vi "niRFUtil FWK Get Driver Version.vi"(8 "error in (no error)":errorcluster, 11 "Registry Key":string[](array[string])=["SOFTWARE\\National Instruments\\NI-RFSA\\Run-Time", "SOFTWARE\\National Instruments\\VST\\NI-RFSA Support\\Current Version", "SOFTWARE\\National Instruments\\VST20\\NI-RFSA Support\\Current Version"]) -> (0 "error out":errorcluster, 1 "Major Version":i32, 2 "VersionString":string, 3 "Version":string, 4 "Minor Version":i32)   [LabVIEW 2015, in "niRFUtil.lvlib"]
uses:
  niRFUtil.lvlib
  <vilib>/registry/registry.llb/Registry RtKey.ctl
  <vilib>/registry/registry.llb/Registry SAM.ctl
  <vilib>/registry/registry.llb/Read Registry Value Simple STR.vi
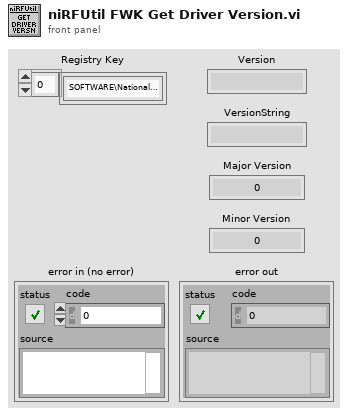
[diagram p1: front panel]
types:
  T1 = typedef "Registry SAM.ctl" = enum32{"KEY_QUERY_VALUE", "KEY_SET_VALUE", "KEY_CREATE_SUB_KEY", "KEY_ENUMERATE_SUB_KEYS", "KEY_NOTIFY", "KEY_CREATE_LINK", "KEY_READ", "KEY_WRITE", "KEY_ALL_ACCESS", "KEY_READ | KEY_WRITE"}
  T2 = typedef "Registry RtKey.ctl" = enum32{"HKEY_CLASSES_ROOT", "HKEY_CURRENT_USER", "HKEY_LOCAL_MACHINE", "HKEY_USERS", "HKEY_PERFORMANCE_DATA", "HKEY_CURRENT_CONFIG", "HKEY_DYN_DATA"}
  T3 = typedef "Registry refnum.ctl" = refnum<k1>
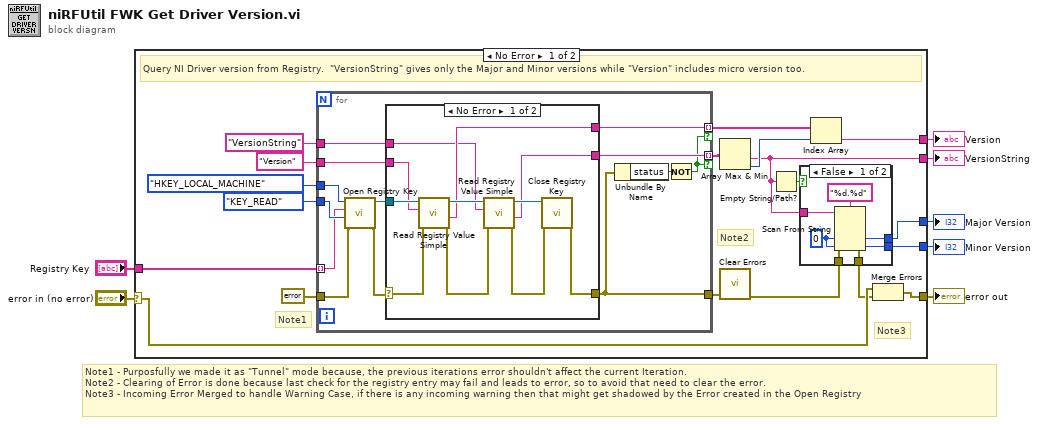
[diagram p0: block diagram]
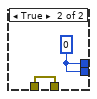
[diagram p2: hidden frame]
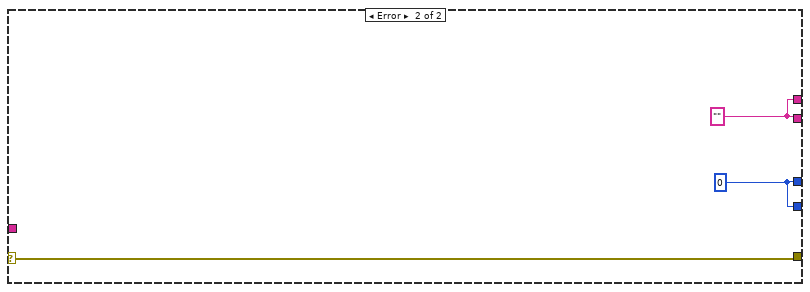
[diagram p4: hidden frame]
diagram:
  # "Note1 - Purposfully we made it as \"Tunnel\" mode because, the previous iterations error shouldn't affect the current Iteration. \nNote2 - Clearing of Error is done because last check for the registry entry may fail and leads to error, so to avoid that need to clear the error.\nNote3 - Incoming Error Merged to handle Warning Case, if there is any incoming warning then that might get shadowed by the Error created in the Open Registry"
  n1 = case shown="No Error" "error in (no error)" {
    selector: "error in (no error)" -> [w17 w63]
    tunnel: [w18 w63] -> w7
    tunnel: [w11 w61] -> w5
    tunnel: [w12 w61] -> w4
    tunnel: [w19 w62] -> w3
    tunnel: [w10 w62] -> w2
    tunnel: "Registry Key" -> [w8 _]
    frame No Error {
      # "Note3"
      # "Note2"
      # "Note1"
      # "Query NI Driver version from Registry.  \"VersionString\" gives only the Major and Minor versions while \"Version\" includes micro version too."
      n2 = for {
        tunnel: Registry_RtKey."HKEY_LOCAL_MACHINE" ("root key (HKEY_LOCAL_MACHINE)") -> [w46]
        tunnel: Registry_SAM."KEY_READ" ("security access mask (KEY_READ | KEY_WRITE)") -> [w45]
        tunnel: "VersionString" ("value") -> [w44]
        tunnel: "Version" ("value") -> [w43]
        tunnel: w8 -> [w41] mode=indexing
        tunnel: [w40] -> w21 mode=indexing if=w36
        tunnel: [w39] -> w15 mode=indexing if=w36
        tunnel: errorcluster {"status"=FALSE, "code"=0, "source"=""} ("error IO") -> [w47]
        tunnel: [w38] -> w26
        n3 = call <vilib>:"Open Registry Key.vi"("error in (no error)"=w47, "security access mask (KEY_READ | KEY_WRITE)"=w45, "subkey"=w41, "root key (HKEY_LOCAL_MACHINE)"=w46) -> ("error out"=w42:errorcluster, "refnum out"=w48:T3)  [unwired: 6 in]
        n4 = case shown="No Error" w42 {
          selector: w42 -> [w50 w60]
          tunnel: w48 -> [w59 _]
          tunnel: [w55 w60] -> w38
          tunnel: [w54 _] -> w40
          tunnel: w44 -> [w52 _]
          tunnel: w43 -> [w51 _]
          tunnel: [w49 _] -> w39
          frame No Error {
            n5 = call-poly <vilib>:"Read Registry Value Simple.vi"("error in (no error)"=w50, "value"=w51, "refnum"=w59) -> ("error out"=w57:errorcluster, "String/Binary data"=w54:string, "refnum out"=w58:T3)  [unwired: 3 in, 1 out]
            n6 = call-poly <vilib>:"Read Registry Value Simple.vi"("error in (no error)"=w57, "value"=w52, "refnum"=w58) -> ("error out"=w53:errorcluster, "String/Binary data"=w49:string, "refnum out"=w56:T3)  [unwired: 3 in, 1 out]
            n7 = call <vilib>:"Close Registry Key.vi"("error in (no error)"=w53, "refnum"=w56) -> ("error out"=w55:errorcluster)  [unwired: 5 in]
          }
          frame Error {
          }
        }
        n8 = Unbundle By Name(w38) -> ("status"=w37:bool)
        n9 = Not(x=w37) -> (.not. x?=w36:bool)
      }
      n10 = Array Max & Min(array=w15) -> (min value=w10:string, min index (indices)=w20:i32)  [unwired: 2 out]
      n11 = call <vilib>:"Clear Errors.vi"("error in (no error)"=w26) -> ("error out"=w14:errorcluster)  [unwired: 5 in, 1 out]
      n12 = Empty String/Path?(string/path=w10) -> (empty?=w9:bool)
      n13 = case shown="False" w9 {
        tunnel: w14 -> [w31 w34]
        tunnel: [w30 w34] -> w13
        tunnel: [w29 w35] -> w12
        tunnel: [w28 w35] -> w11
        tunnel: w10 -> [w27 _]
        frame False {
          w32 = 0 ("initial scan location")
          n14 = Scan From String(format string="%d.%d", input string=w27, error in=w31, default 1=w32, default 2=w32) -> (error out=w30:errorcluster, output 1=w29:i32, output 2=w28:i32)  [unwired: 1 in, 2 out]
        }
        frame True {
          w35 = 0 ("initial scan location")
        }
      }
      n15 = Index Array(array=w21, index=w20) -> (element=w19:string)
      n16 = Merge Errors(w17, w13) -> (w18:errorcluster)
    }
    frame Error {
      w61 = 0 ("initial scan location")
      w62 = "" ("String/Binary data")
    }
  }
  "error out" <- w7
  "Minor Version" <- w5
  "Major Version" <- w4
  "VersionString" <- w2
  "Version" <- w3
